vi "COM_Write&Read.vi"(7 "Read?":bool=TRUE, 8 "error in (no error)":errorcluster, 9 "String":string, 10 "wait ms":i32=100, 11 "VISA Refnum in":refnum<visa-resource-name>) -> (0 "error out":errorcluster, 2 "read buffer":string, 3 "VISA Refnum out":refnum<visa-resource-name>)   [LabVIEW 2013]
uses:
  <vilib>/Instr/_visa.llb/VISA Flush IO Buffer Mask.ctl
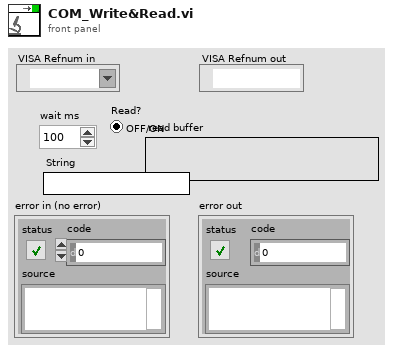
[diagram p1: front panel]
types:
  T1 = typedef "VISA Flush IO Buffer Mask.ctl" = u16
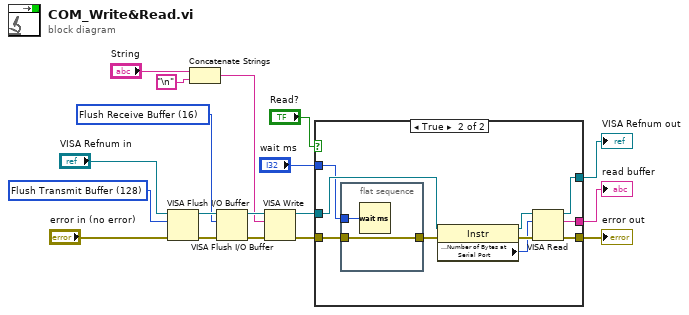
[diagram p0: block diagram]
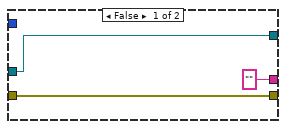
[diagram p2: hidden frame]
diagram:
  w8 = T1 16 items=["Flush Receive Buffer"=16, "Write Transmit Buffer to Device"=32, "Flush Receive Buffer (No I/O)"=64, "Flush Transmit Buffer"=128] ("Mask")
  w9 = T1 128 items=["Flush Receive Buffer"=16, "Write Transmit Buffer to Device"=32, "Flush Receive Buffer (No I/O)"=64, "Flush Transmit Buffer"=128] ("Mask")
  n1 = VISA Flush I/O Buffer(VISA resource name="VISA Refnum in", mask (16)=w9, error in (no error)="error in (no error)") -> (VISA resource name out=w10:refnum<visa-resource-name>, error out=w6:errorcluster)
  n2 = Concatenate Strings("String", "\n") -> (w2:string)
  n3 = VISA Flush I/O Buffer(VISA resource name=w10, mask (16)=w8, error in (no error)=w6) -> (VISA resource name out=w7:refnum<visa-resource-name>, error out=w5:errorcluster)
  n4 = VISA Write(VISA resource name=w7, write buffer=w2, error in (no error)=w5) -> (VISA resource name out=w15:refnum<visa-resource-name>, error out=w13:errorcluster)  [unwired: 1 out]
  n5 = case shown="True" "Read?" {
    tunnel: ["" ("read buffer") w31] -> w18
    tunnel: [w20 w30] -> w17
    tunnel: [w21 w29] -> w16
    tunnel: w15 -> [w21 w26]
    tunnel: "wait ms" -> [_ w25]
    tunnel: w13 -> [w20 w23]
    frame False {
    }
    frame True {
      n6 = flat-sequence {
        tunnel: w25 -> [w33]
        tunnel: [w32] -> w24
        tunnel: w23 -> [w32]
        frame #0 {
          n7 = Wait (ms)(milliseconds to wait=w33) -> ()  [unwired: 1 out]
        }
      }
      n8 = property class="Instr"(reference=w26, error in=w24) -> (reference out=w27:refnum<visa-resource-name>, error out=w28:errorcluster, "Serial Settings:Number of Bytes at Serial Port"=w22:u32)
      n9 = VISA Read(VISA resource name=w27, byte count=w22, error in (no error)=w28) -> (VISA resource name out=w29:refnum<visa-resource-name>, read buffer=w31:string, error out=w30:errorcluster)  [unwired: 1 out]
    }
  }
  "read buffer" <- w18
  "error out" <- w17
  "VISA Refnum out" <- w16
